vi "Scope.vi"(10 "Label":string, 11 "Wfm":waveform(dbl)[](array[waveform])) -> ()   [LabVIEW 2019, in "DSP.lvclass"]
uses:
  DSP.lvclass
panel:
  in  "index":i32
  out "PS Waveform":waveform(dbl)(graph)
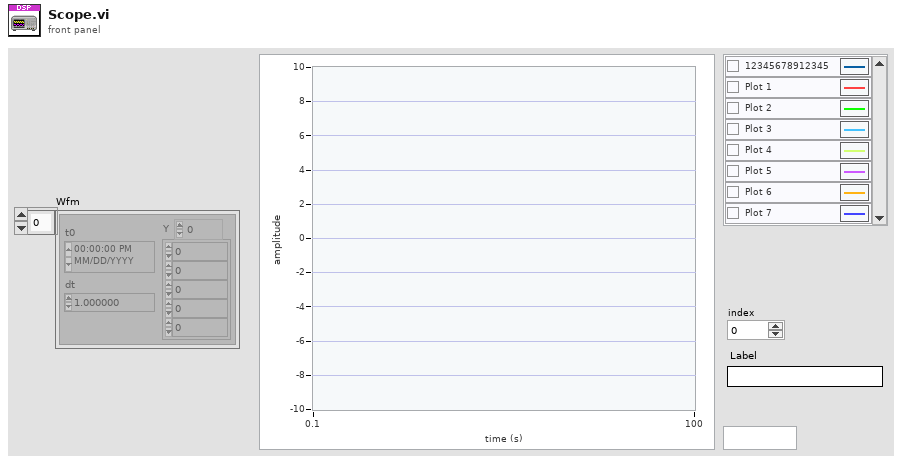
[diagram p1: front panel]
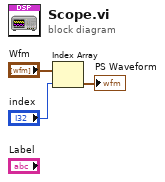
[diagram p0: block diagram]
diagram:
  n1 = Index Array(array="Wfm", index="index") -> (element=→"PS Waveform":waveform(dbl))
